vi "Capacitor to Sweep to Register to Write.vi"(8 "error in (no error)":errorcluster, 11 "Toggle 6 in":refnum<class "Toggle 6.lvclass">) -> (0 "error out":errorcluster, 1 "Cap Value Array":cluster{"Register Number":u32, "Value":dbl}[](array[cluster]), 2 "Cap Register Array":T1[](array[typedef]), 3 "Toggle 6 out":refnum<class "Toggle 6.lvclass">)   [LabVIEW 2020, in "Toggle 6.lvclass"]
uses:
  Toggle 6.lvclass
  Controls/Register to Write.ctl
  PIC-device/PIC-Device.lvclass
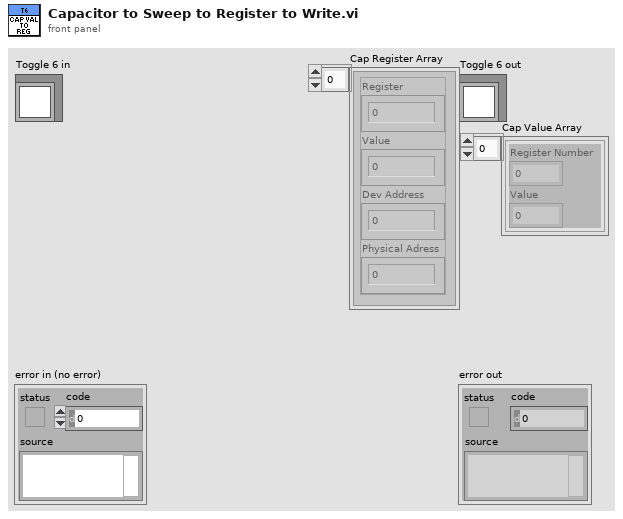
[diagram p1: front panel]
types:
  T1 = typedef "PIC-Device.lvclass/Register to Write.ctl" = cluster{"Register":u32, "Value":u32, "Dev Address":u32, "Physical Adress":u32}
  T2 = typedef "Toggle 6.lvclass/Parameter Cluster.ctl" = cluster{"Enable":bool, "Register Number":u32, "Use Array":bool, "Array":dbl[], "To From Cluster":cluster{"From":dbl, "To":dbl, "Step":dbl}}
  T3 = typedef "Toggle 6.lvclass/Capacitor register.ctl" = cluster{"Register":u32, "Beam":dbl, "Trimmer":dbl}
  T4 = cluster{"Register Number":u32, "Numeric Control":dbl}
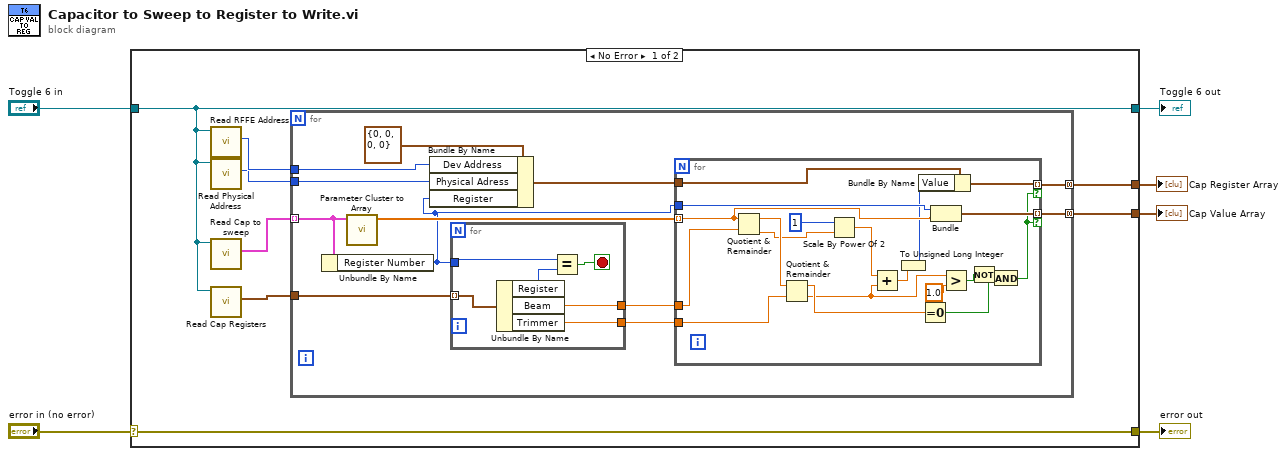
[diagram p0: block diagram]
diagram:
  n1 = case shown="No Error" "error in (no error)" {
    selector: "error in (no error)" -> [w14 w54]
    tunnel: [w14 w54] -> w5
    tunnel: [w11 w53] -> w3
    tunnel: "Toggle 6 in" -> [w11 w53]
    tunnel: [w8 _] -> w2
    tunnel: [w7 _] -> w1
    frame No Error {
      n2 = call-dynamic "Read RFFE Address.vi"("Toggle 6 in"=w11) -> ("RFFE Adress"=w10:u32)  [unwired: 8 in, 2 out]
      n3 = call-dynamic "Read Physical Address.vi"("Toggle 6 in"=w11) -> ("Physical Adress"=w9:u32)  [unwired: 9 in, 1 out]
      n4 = call-dynamic "Read Cap to sweep.vi"("Toggle 6 in"=w11) -> ("Cap to sweep"=w13:T2[])  [unwired: 9 in, 1 out]
      n5 = call-dynamic "Read Cap Registers.vi"("Toggle 6 in"=w11) -> ("Cap Registers"=w12:T3[])  [unwired: 9 in, 1 out]
      n6 = for {
        tunnel: w13 -> [w26] mode=indexing
        tunnel: w12 -> [w25]
        tunnel: w10 -> [w20]
        tunnel: w9 -> [w19]
        tunnel: [w16] -> w8 mode=concatenating
        tunnel: [w15] -> w7 mode=concatenating
        n7 = Unbundle By Name(w26) -> ("Register Number"=w17:u32)
        n8 = call "Parameter Cluster to Array.vi"("Parameter Cluster"=w26) -> ("Array"=w24:dbl[])  [unwired: 10 in]
        n9 = Bundle By Name(cluster=T1 {"Register"=0, "Value"=0, "Dev Address"=0, "Physical Adress"=0} ("Register to Write"), "Dev Address"=w20, "Physical Adress"=w19, "Register"=w17) -> (w18:T1)
        n10 = for {
          tunnel: w17 -> [w50]
          tunnel: w25 -> [w52] mode=indexing
          tunnel: [w48] -> w23
          tunnel: [w47] -> w22
          stop <- w49 stop-if-true
          n11 = Unbundle By Name(w52) -> ("Register"=w51:u32, "Beam"=w48:dbl, "Trimmer"=w47:dbl)
          n12 = Equal?(x=w50, y=w51) -> (x = y?=w49:bool)
        }
        n13 = for {
          tunnel: w24 -> [w39] mode=indexing
          tunnel: w23 -> [w46]
          tunnel: w22 -> [w44]
          tunnel: w18 -> [w37]
          tunnel: w17 -> [w40]
          tunnel: [w38] -> w15 mode=indexing if=w29
          tunnel: [w34] -> w16 mode=indexing if=w29
          n14 = Quotient & Remainder(x=w39, y=w46) -> (x-y*floor(x/y)=w45:dbl, floor(x/y)=w42:dbl)
          n15 = Quotient & Remainder(x=w45, y=w44) -> (x-y*floor(x/y)=w33:dbl, floor(x/y)=w32:dbl)
          n16 = Scale By Power Of 2(n=i16 1, x=w42) -> (x*2^n=w41:dbl)
          n17 = Add(x=w41, y=w32) -> (x+y=w36:dbl)
          n18 = To Unsigned Long Integer(number=w36) -> (unsigned 32bit integer=w35:u32)
          n19 = Bundle By Name(cluster=w37, "Value"=w35) -> (w34:T1)
          n20 = Equal To 0?(x=w33) -> (x = 0?=w27:bool)
          n21 = Bundle("Register Number"=w40, "Numeric Control"=w39) -> (w38:T4)  [unwired: 1 in]
          n22 = Greater?(x=w32, y=1.0) -> (0:w30:bool)
          n23 = Not(x=w30) -> (.not. x?=w28:bool)
          n24 = And(x=w28, y=w27) -> (x .and. y?=w29:bool)
        }
      }
    }
    frame Error {
    }
  }
  "error out" <- w5
  "Toggle 6 out" <- w3
  "Cap Register Array" <- w2
  "Cap Value Array" <- w1
